vi "Ultrasonic.vi"(1 "State":enum16{"Start", "Run", "Finish"}(ring)) -> (0 "Distance (in)":dbl)   [LabVIEW 2014]
uses:
  <vilib>/Rock Robotics/SystemInterfaces/AI/FPGA_AIChannel.ctl
  <vilib>/Rock Robotics/WPI/Ultrasonic/WPI_SonarMB1010AnalogOpen.vi
  <vilib>/Rock Robotics/WPI/Ultrasonic/WPI_SonarMB1010AnalogGetRange.vi
  <vilib>/Rock Robotics/Network Tables/SD Write Number.vi
  <vilib>/Rock Robotics/WPI/Ultrasonic/WPI_SonarMB1010AnalogClose.vi
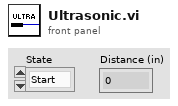
[diagram p1: front panel]
types:
  T1 = typedef "FPGA_AIChannel.ctl" = enum8{"AI 0", "AI 1", "AI 2", "AI 3", "AI MXP 0", "AI MXP 1", "AI MXP 2", "AI MXP 3", "Invalid"}
  T2 = typedef "WPI_SonarMB1010AnalogDeviceRef.ctl" = cluster{"AIDeviceRef":T3, "Scaling factor (V/in)":dbl, "Average Bits":u8}
  T3 = typedef "WPI_AnalogChannelDevRef.ctl" = cluster{"DevStatus":errorcluster, "Controller":T4, "Analog Channel":T1}
  T4 = typedef "FPGA_TypedefAnalogModule.ctl" = enum16{"Controller 1"}
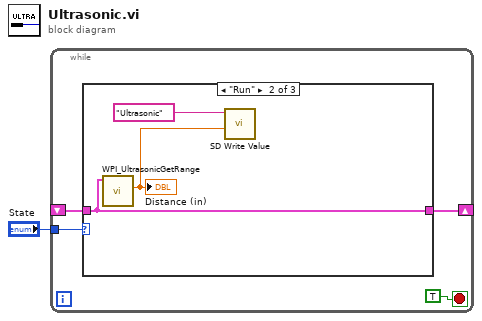
[diagram p0: block diagram]
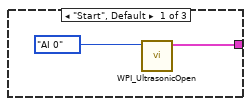
[diagram p2: hidden frame]
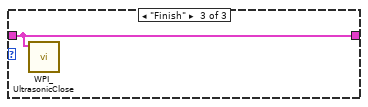
[diagram p3: hidden frame]
diagram:
  n1 = while {
    tunnel: "State" -> [w5]
    shift-right: [w3] -> _
    shift-left: _ -> [w2]
    stop <- TRUE stop-if-true
    n2 = case shown="\"Run\"" w5 {
      tunnel: [w7 w10 w11] -> w3
      tunnel: w2 -> [_ w10 w11]
      frame "Start", Default {
        n3 = call-poly <vilib>:"WPI_UltrasonicOpen.vi"("Analog Channel"=FPGA_AIChannel."AI 0") -> ("SonarMB1010AnalogDevRef"=w7:T2)  [unwired: 9 in, 1 out]
      }
      frame "Run" {
        n4 = call-poly <vilib>:"WPI_UltrasonicGetRange.vi"("SonarMB1010AnalogDevRef"=w10) -> ("Distance"=w9:dbl)  [unwired: 8 in, 2 out]
        "Distance (in)" <- w9
        n5 = call-poly <vilib>:"SD Write Value.vi"("Numeric"=w9, "Name"="Ultrasonic") -> ()  [unwired: 8 in, 2 out]
      }
      frame "Finish" {
        n6 = call-poly <vilib>:"WPI_UltrasonicClose.vi"("SonarMB1010AnalogDevRef"=w11) -> ()  [unwired: 10 in, 1 out]
      }
    }
  }
